vi "String_to_Ch_names.vi"(0 "Spreadsheet string":string) -> (1 "Ch names":string[](array[string]), 2 "Title length (Bytes)":i32, 3 "Title Rows Found?":bool, 4 "String After names":string)   [LabVIEW 2020]
panel:
  out "Data length":i32
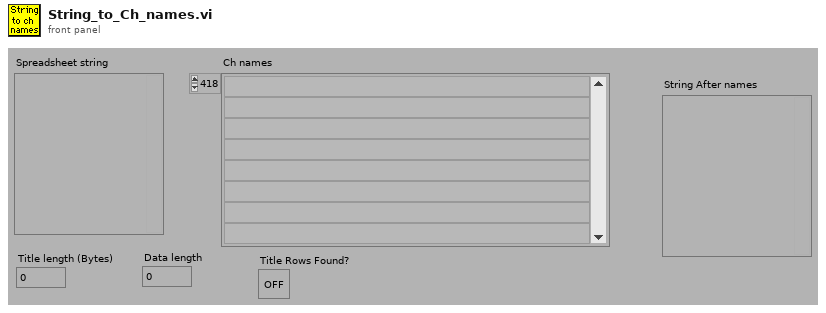
[diagram p1: front panel]
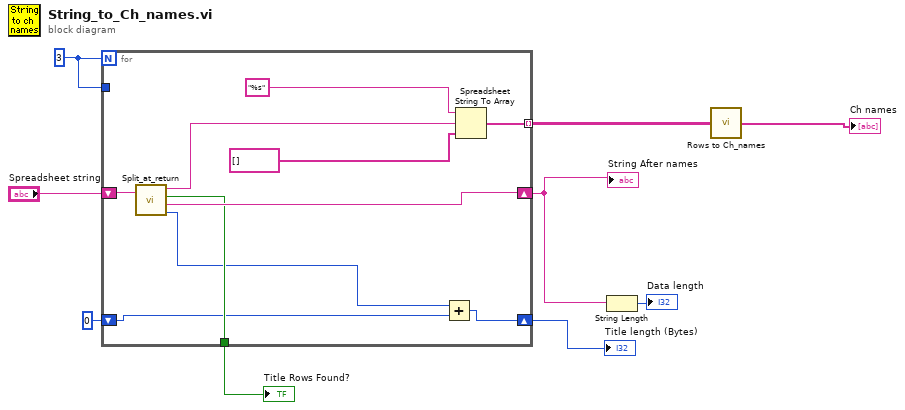
[diagram p0: block diagram]
diagram:
  w9 = 3
  n1 = for {
    N: w9 -> [_]
    shift-right: [w16] -> w7
    shift-left: "Spreadsheet string" -> [w17]
    tunnel: w9 -> [_]
    tunnel: [w14] -> w1
    tunnel: [w15] -> w6 mode=indexing
    shift-right: [w12] -> w3
    shift-left: 0 -> [w13]
    n2 = call "Split_at_return.vi"("String"=w17) -> ("before substring"=w11:string, "Matched?"=w14:bool, "after substring"=w16:string, "offset past match"=w10:i32)  [unwired: 1 in]
    n3 = Add(x=w10, y=w13) -> (x+y=w12:i32)
    n4 = Spreadsheet String To Array(format string="%s", spreadsheet string=w11, array type (2D Dbl)=string[] []) -> (array=w15:string[])  [unwired: 1 out]
  }
  "Title length (Bytes)" <- w3
  "String After names" <- w7
  "Title Rows Found?" <- w1
  n5 = String Length(string=w7) -> (length=→"Data length":i32)
  n6 = call "Rows to Ch_names.vi"("array type (2D Dbl)"=w6) -> ("Array"=→"Ch names":string[])
